vi "GET Request.vi"(8 "error in (no error)":errorcluster, 10 "Path (after URL)":string, 11 "EnVision REST in":refnum<class "EnVision REST.lvclass">) -> (0 "error out":errorcluster, 1 "Status Code":u16, 2 "Response":string, 3 "EnVision REST out":refnum<class "EnVision REST.lvclass">)   [LabVIEW 2018, in "EnVision REST.lvlib" / "EnVision REST.lvclass"]
uses:
  EnVision REST.lvclass
  EnVision REST.lvclass/EnVision REST.ctl
  <vilib>/addons/_JKI.lib/REST Client/classes/REST Client/REST Client.lvclass
  PPLs/REST Interface/Parent/REST Interface.lvlibp/REST Interface.lvclass
  C:/Projects/LabVIEW/PPLs/REST Interface/Parent/REST Interface.lvlibp/REST Interface.lvclass
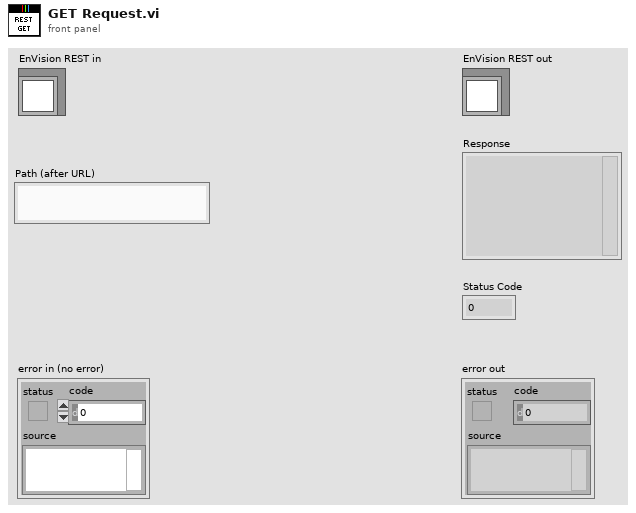
[diagram p1: front panel]
types:
  T1 = typedef "REST Interface.lvlibp/REST Client.lvlib/REST Client.lvclass/HTTP Header.ctl" = cluster{"header":string, "value":string}
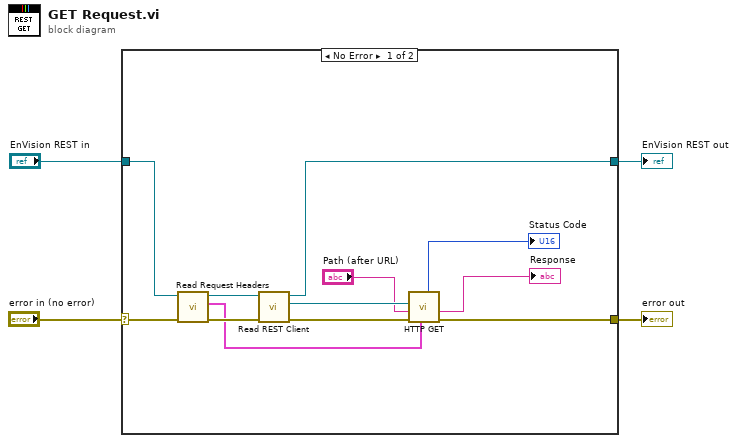
[diagram p0: block diagram]
diagram:
  n1 = case shown="No Error" "error in (no error)" {
    selector: "error in (no error)" -> [w8 w18]
    tunnel: [w10 w18] -> w3
    tunnel: [w16 w17] -> w2
    tunnel: "EnVision REST in" -> [w9 w17]
    frame No Error {
      n2 = call "Read Request Headers.vi"("error in (no error)"=w8, "REST Interface in"=w9) -> ("error out"=w7:errorcluster, "Request Headers"=w5:T1[], "REST Interface out"=w6:refnum<class "EnVision REST.lvclass">)  [unwired: 7 in]
      n3 = call "Read REST Client.vi"("error in (no error)"=w7, "EnVision REST in"=w6) -> ("error out"=w15:errorcluster, "REST Client.lvlib:REST Client.lvclass"=w14:refnum<class "REST Client.lvclass">, "EnVision REST out"=w16:refnum<class "EnVision REST.lvclass">)  [unwired: 7 in]
      n4 = call-dynamic "HTTP GET.vi"("request specific headers"=w5, "error in (no error)"=w15, "Path"="Path (after URL)", "REST Client in"=w14) -> ("error out"=w10:errorcluster, "Response body"=→"Response":string, "Status Code"=→"Status Code":u16)  [unwired: 2 in, 3 out]
    }
    frame Error {
    }
  }
  "error out" <- w3
  "EnVision REST out" <- w2
